vi "DAQ@Wait__Parameter.vi"(1 "ParamterIn":string) -> (0 "ParamterOut":string)   [LabVIEW 2020]
panel:
  in  "DAQName":string(combo)
  in  "Confirm":bool
  # "DAQ@Wait $DAQNAME"
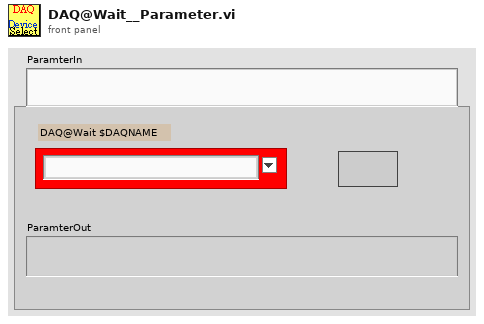
[diagram p1: front panel]
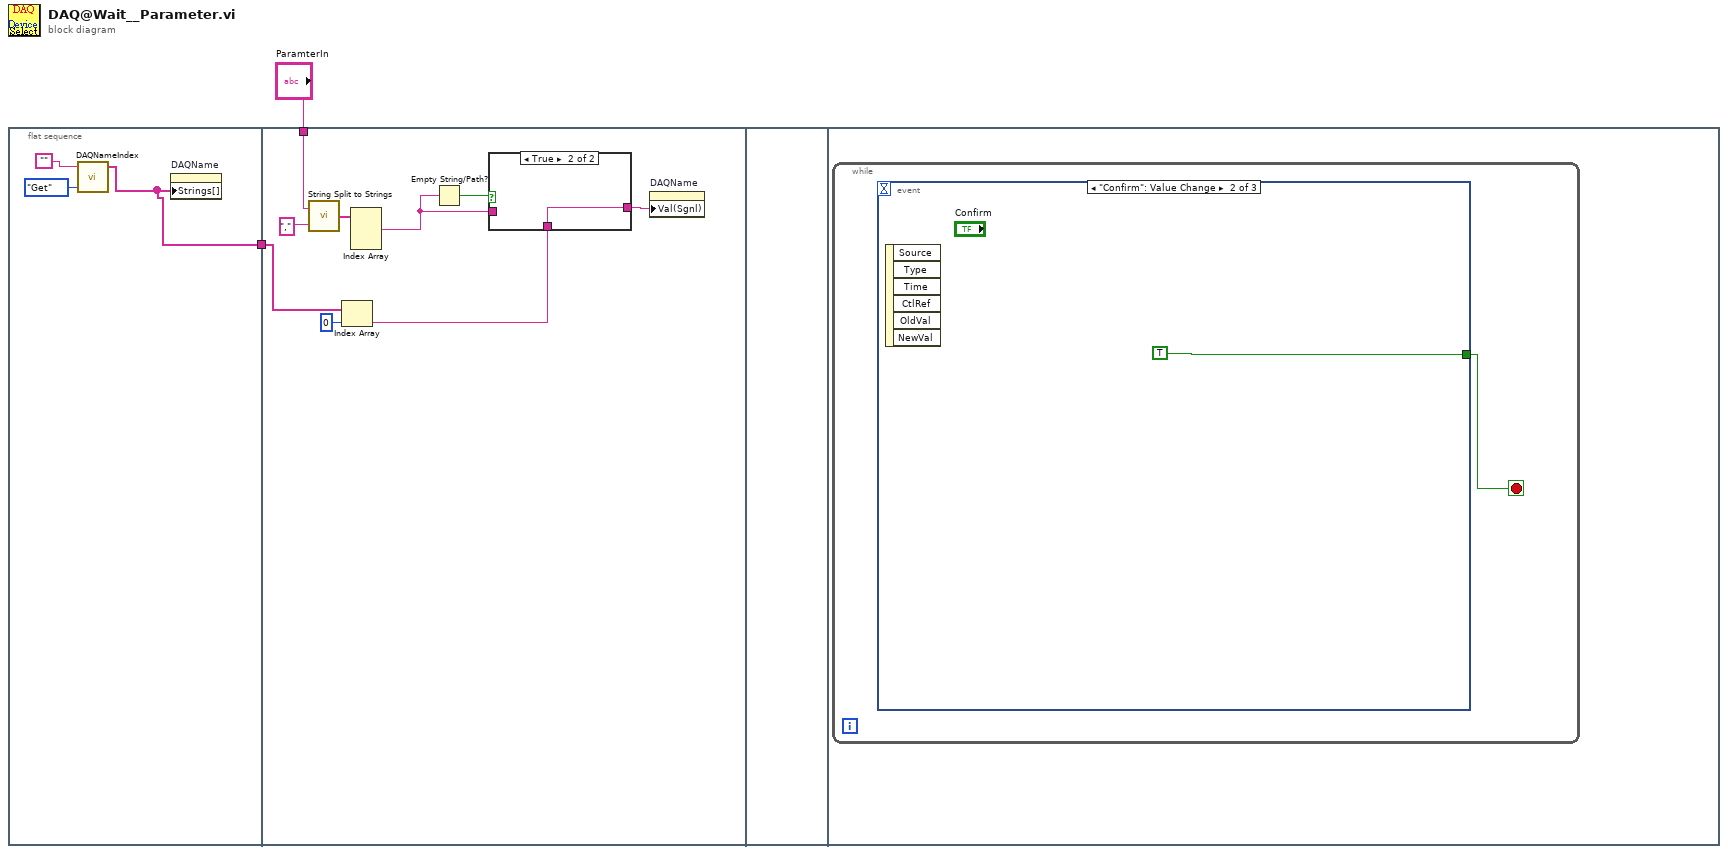
[diagram p0: block diagram]
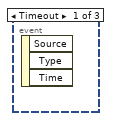
[diagram p3: hidden frame]
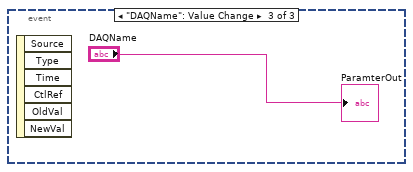
[diagram p4: hidden frame]
diagram:
  n1 = flat-sequence {
    tunnel: [w3] -> w1
    tunnel: "ParamterIn" -> [w12]
    tunnel: w1 -> [w8]
    frame #0 {
      n2 = call "DAQNameIndex.vi"("OP"=enum16{"Get", "Update", "Init"}."Get", "DAQName"="") -> ("DAQList"=w3:string[])  [unwired: 1 in, 2 out]
      n3 = property on="DAQName" class="CmbBox"("Strings[]"=w3) -> ()  [unwired: 2 in, 2 out]
    }
    frame #1 {
      n4 = call "String Split to Strings.vi"("search string/char (-)"=",", "String"=w12) -> ("Array"=w14:string[])
      n5 = Index Array(array=w8, index=0) -> (element=w6:string)
      n6 = Index Array(array=w14) -> (element #1=w10:string)  [unwired: 3 in, 2 out]
      n7 = Empty String/Path?(string/path=w10) -> (empty?=w11:bool)
      n8 = case shown="True" w11 {
        tunnel: w10 -> [w15 _]
        tunnel: [w15 w16] -> w9
        tunnel: w6 -> [_ w16]
        frame False {
        }
        frame True {
        }
      }
      n9 = property on="DAQName" class="CmbBox"("Val(Sgnl)"=w9) -> ()  [unwired: 2 in, 2 out]
    }
    frame #2 {
    }
    frame #3 {
      n10 = while {
        stop <- w17 stop-if-true
        n11 = event shown="[1] \"Confirm\": Value Change" {
          selector: _ -> [_ _ _]
          dyn-events: _ -> [_ _ _]
          timeout: _ -> [_ _ _]
          tunnel: [_ TRUE _] -> w17
          event Timeout {
            n12 = event-data() -> ()  [unwired: 1 in, 3 out]
          }
          event "Confirm": Value Change {
            n13 = event-data() -> ()  [unwired: 1 in, 6 out]
          }
          event "DAQName": Value Change {
            n14 = event-data() -> ()  [unwired: 1 in, 6 out]
            "ParamterOut" <- "DAQName"
          }
        }
      }
    }
  }
